vi "Configure Control AI Range(Volt Sqrt).vi"(0 "VISA resource name":refnum<visa-resource-name>, 1 "Unit No. (0)":i32 min=0 max=6, 3 "Range And Span":T3={"Volt Range (4 : 2V)"=4, "Enable Span (False)"=FALSE, "Lower Span (2.0000)"=-2.0, "Upper Span (2.0000)"=2.0, "Bias (0)"=0.0} {"Upper Span (2.0000)" min=-99999.0 max=99999.0 step=1.0 format="%_5g"; "Lower Span (2.0000)" min=-99999.0 max=99999.0 step=1.0 format="%_5g"; "Volt Range (4 : 2V)" items=["20mV", "60mV", "200mV", "1V", "2V", "6V", "20V", "50V"]}, 4 "Module No.(0)":i32 min=0 max=9, 5 "AI No.(1)":i32=1 min=1 max=2, 6 "Low cut":T1 {"Output (0: Zero)" items=["Zero", "Linear"]; "Low-cut (0.0)" min=0.0 max=5.0}, 7 "error in (no error)":errorcluster, 8 "Scaling":T2={"Floating Point Position (2)"=2, "Lower Scaling (0)"=0.0, "Upper Scaling (10000)"=100.0, "Unit Character (\"\")"=""} {"Upper Scaling (10000)" format="%_6g"; "Lower Scaling (0)" format="%_6g"; "Floating Point Position (2)" min=0 max=5 step=1}) -> (20 "VISA resource name out":refnum<visa-resource-name>, 21 "AI No.":i32, 24 "Unit No.":i32, 25 "Module No.":i32, 27 "error out":errorcluster)   [LabVIEW 2020, in "Yokogawa GX Series.lvlib"]
doc: "Set Volt range of AI channel in PID module.\n\nCommand: SCtrlRangeAI"
uses:
  <instrlib>/Yokogawa GX Series/Yokogawa GX Series.lvlib
  <instrlib>/Yokogawa GX Series/Private/Volt Range.vi
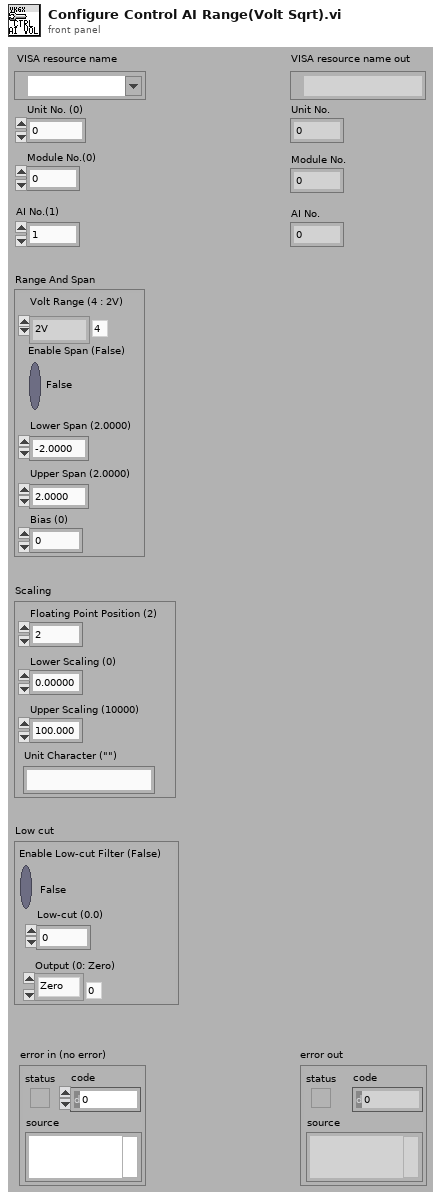
[diagram p1: front panel]
types:
  T1 = cluster{"Enable Low-cut Filter (False)":bool, "Low-cut (0.0)":dbl, "Output (0: Zero)":u16}
  T2 = cluster{"Floating Point Position (2)":i32, "Lower Scaling (0)":dbl, "Upper Scaling (10000)":dbl, "Unit Character (\"\")":string}
  T3 = cluster{"Volt Range (4 : 2V)":i32, "Enable Span (False)":bool, "Lower Span (2.0000)":dbl, "Upper Span (2.0000)":dbl, "Bias (0)":dbl}
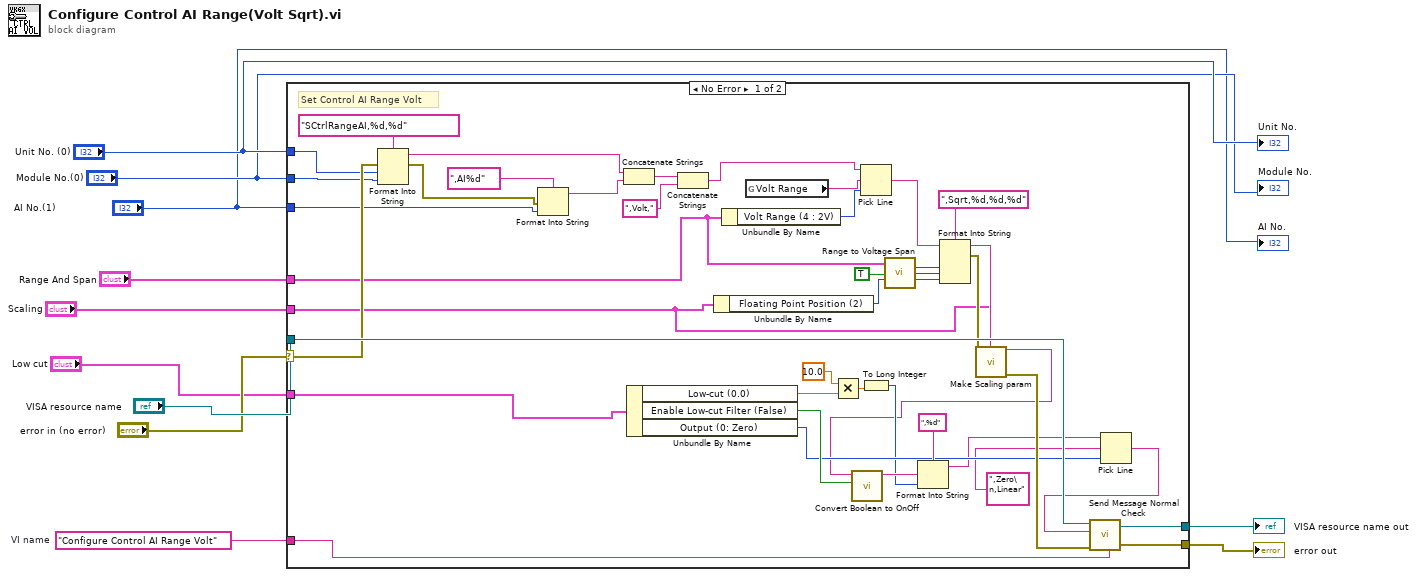
[diagram p0: block diagram]
diagram:
  w7 = "Configure Control AI Range Volt"  # VI name
  n1 = case shown="No Error" "error in (no error)" {
    selector: "error in (no error)" -> [w50 w55]
    tunnel: [w54 w56] -> w11
    tunnel: [w53 w55] -> w10
    tunnel: "VISA resource name" -> [w52 w56]
    tunnel: w7 -> [w49 _]
    tunnel: "Unit No. (0)" -> [w48 _]
    tunnel: "Module No.(0)" -> [w47 _]
    tunnel: "AI No.(1)" -> [w45 _]
    tunnel: "Range And Span" -> [w29 _]
    tunnel: "Scaling" -> [w26 _]
    tunnel: "Low cut" -> [w14 _]
    frame No Error {
      # "Set Control AI Range Volt"
      n2 = Format Into String(format string="SCtrlRangeAI,%d,%d", error in=w50, w48, w47) -> (resulting string=w43:string, error out=w44:errorcluster)  [unwired: 1 in]
      n3 = Format Into String(format string=",AI%d", error in=w44, w45) -> (resulting string=w42:string)  [unwired: 1 in, 1 out]
      n4 = Concatenate Strings(w43, w42) -> (w41:string)
      n5 = Unbundle By Name(w14) -> ("Low-cut (0.0)"=w17:dbl, "Enable Low-cut Filter (False)"=w23:bool, "Output (0: Zero)"=w22:u16)
      n6 = Concatenate Strings(w41, ",Volt,") -> (w31:string)
      n7 = Unbundle By Name(w26) -> ("Floating Point Position (2)"=w33:i32)
      n8 = Unbundle By Name(w29) -> ("Volt Range (4 : 2V)"=w39:i32)
      n9 = global read "Volt Range.vi" "Volt Range"() -> (w30:string)
      n10 = Multiply(x=10.0, y=w17) -> (x*y=w16:dbl)
      n11 = Pick Line(string ("")=w31, multi-line string=w30, line index=w39) -> (output string=w28:string)
      n12 = To Long Integer(number=w16) -> (32bit integer=w15:i32)
      n13 = call <instrlib>:"Range to Voltage Span.vi"("Range And Span"=w29, "Scaling? (False)"=TRUE, "Floating Point Position (2)"=w33) -> ("Lower Span"=w38:i32, "Upper Span"=w37:i32, "Bias"=w36:i32)  [unwired: 5 in, 5 out]
      n14 = Format Into String(format string=",Sqrt,%d,%d,%d", initial string=w28, w38, w37, w36) -> (resulting string=w32:string, error out=w34:errorcluster)  [unwired: 1 in]
      n15 = call <instrlib>:"Make Scaling param.vi"("String (\"\")"=w32, "Scaling"=w26, "error in (no error)"=w34) -> ("String After"=w13:string, "error out"=w25:errorcluster)  [unwired: 11 in]
      n16 = call <instrlib>:"Convert Boolean to OnOff.vi"("On/Off"=w23, "Initial String (\"\")"=w13) -> ("Resulting String"=w21:string)  [unwired: 9 in]
      n17 = Format Into String(format string=",%d", initial string=w21, w15) -> (resulting string=w20:string)  [unwired: 1 in, 1 out]
      n18 = Pick Line(string ("")=w20, multi-line string=",Zero\n,Linear", line index=w22) -> (output string=w12:string)
      n19 = call <instrlib>:"Send Message Normal Check.vi"("Source (\"\")"=w49, "error in (no error)"=w25, "Send Message (\"\")"=w12, "VISA resource name"=w52) -> ("error out"=w53:errorcluster, "VISA resource name out"=w54:refnum<visa-resource-name>)  [unwired: 2 in, 4 out]
    }
    frame Error {
    }
  }
  "error out" <- w10
  "VISA resource name out" <- w11
  "Unit No." <- "Unit No. (0)"
  "Module No." <- "Module No.(0)"
  "AI No." <- "AI No.(1)"
